vi "SLM_Control_Sample.vi"() -> ()   [LabVIEW 2018]
panel:
  in  "STOP button":bool
  out "Dffraction image":picture caption="Diffraction image"
  out "LG Beam image":picture
  out "Cylindrical lense image":picture caption="Cylindrical Lens image"
  out "Axicon image":picture
  out "Target image":picture
  out "Correction image":picture
  out "CGH image":picture caption="Tiled CGH image / Target image"
  out "Fresnel Lens image":picture
  out "2nd Display(LCOS) image":picture
  in  "?":T1(tab)
  in  "CGH  ON / OFF":bool=TRUE
  in  "LCOS type":string(combo)="X15223 series"
  in  "Corection image address":path
  in  "Target image address":path
  in  "Repetition Number":u32=100
  in  "Slip":i32
  in  "Cylindrical Lens":bool=TRUE
  in  "Cylindrical Focus/mm":i32=1000
  in  "WaveFront":bool=TRUE
  in  "Fresnel Lens":bool=TRUE
  in  "LUT":bool
  in  "2π Signal Level (0-255)":u8=210
  in  "Fresnel Focus/mm":i32=1000
  in  "Wave length/nm":u32=532
  out "Wave length/nm":u32=532
  in  "Mode Select":enum32{"Row", "Column"}(radio)
  in  "Rotation degree":dbl
  in  "Axicon Lens":bool=TRUE
  in  "Top level / πrad.":dbl=4.0
  in  "LG Beam":bool=TRUE
  in  "m":u32=1
  in  "p":u32=1
  in  "Diffraction":bool=TRUE
  in  "Mode Select2":enum32{"Row", "Column"}(radio)
  in  "gradation width":u32=1
  in  "gradation number":u32=2
  in  "Flip image":i32(listbox)
  in  "Beam size / mm":dbl
  in  "Additional phase mask (2πrad. at 0-255level) 2":path
  in  "Additional phase combination mode\nComplex amplitude / Amplitude 2":bool
  in  "Save 2nd Display image button":bool
  in  "Additional phase combination mode\nComplex amplitude / Amplitude 1":bool=TRUE
  in  "Monitor mumber":i32=2
  in  "Y PixelShift":i32
  in  "X PixelShift":i32
  in  "Additional phase mask (2πrad. at 0-255level) 1":path
  in  "Coef._2":bool=TRUE
  in  "Coef._2":dbl(slide)=1.0 scale=-10.0..10.0
  in  "m_2":i32=1
  in  "n_2":i32=1
  in  "diameter / mm":dbl=10.0 min=1.0
  in  "Coef._1":dbl(slide)=1.0 scale=-10.0..10.0
  in  "Zernike":bool=TRUE
  out "Zernike":picture caption="Zernike image"
  in  "n_1":i32=1
  in  "m_1":i32=-1
  in  "Coef._1":bool=TRUE
  # "Sample code for\nLabVIEW"
  # "Basic Setting Parameter"
  # "LCOS-SLM"
  # "If a null address was input , all 0 pattern will appear."
  # "Target image"
  # "Corection"
  # "CGH"
  # "LCOS display settings"
  # "After press the STOP button, the BMP data save dialog will open."
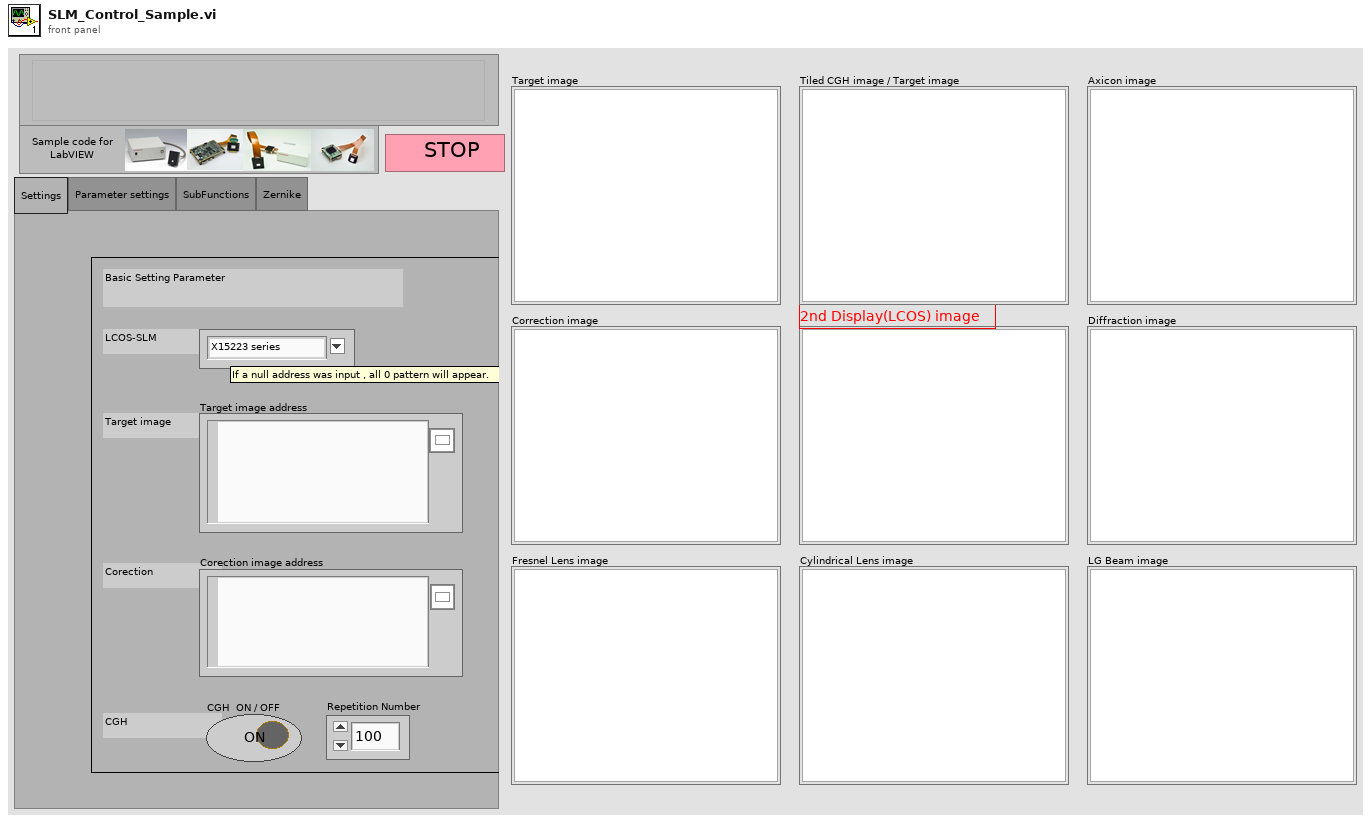
[diagram p1: front panel]
types:
  T1 = enum32{"Settings", "Parameter settings", "SubFunctions", "Zernike"}
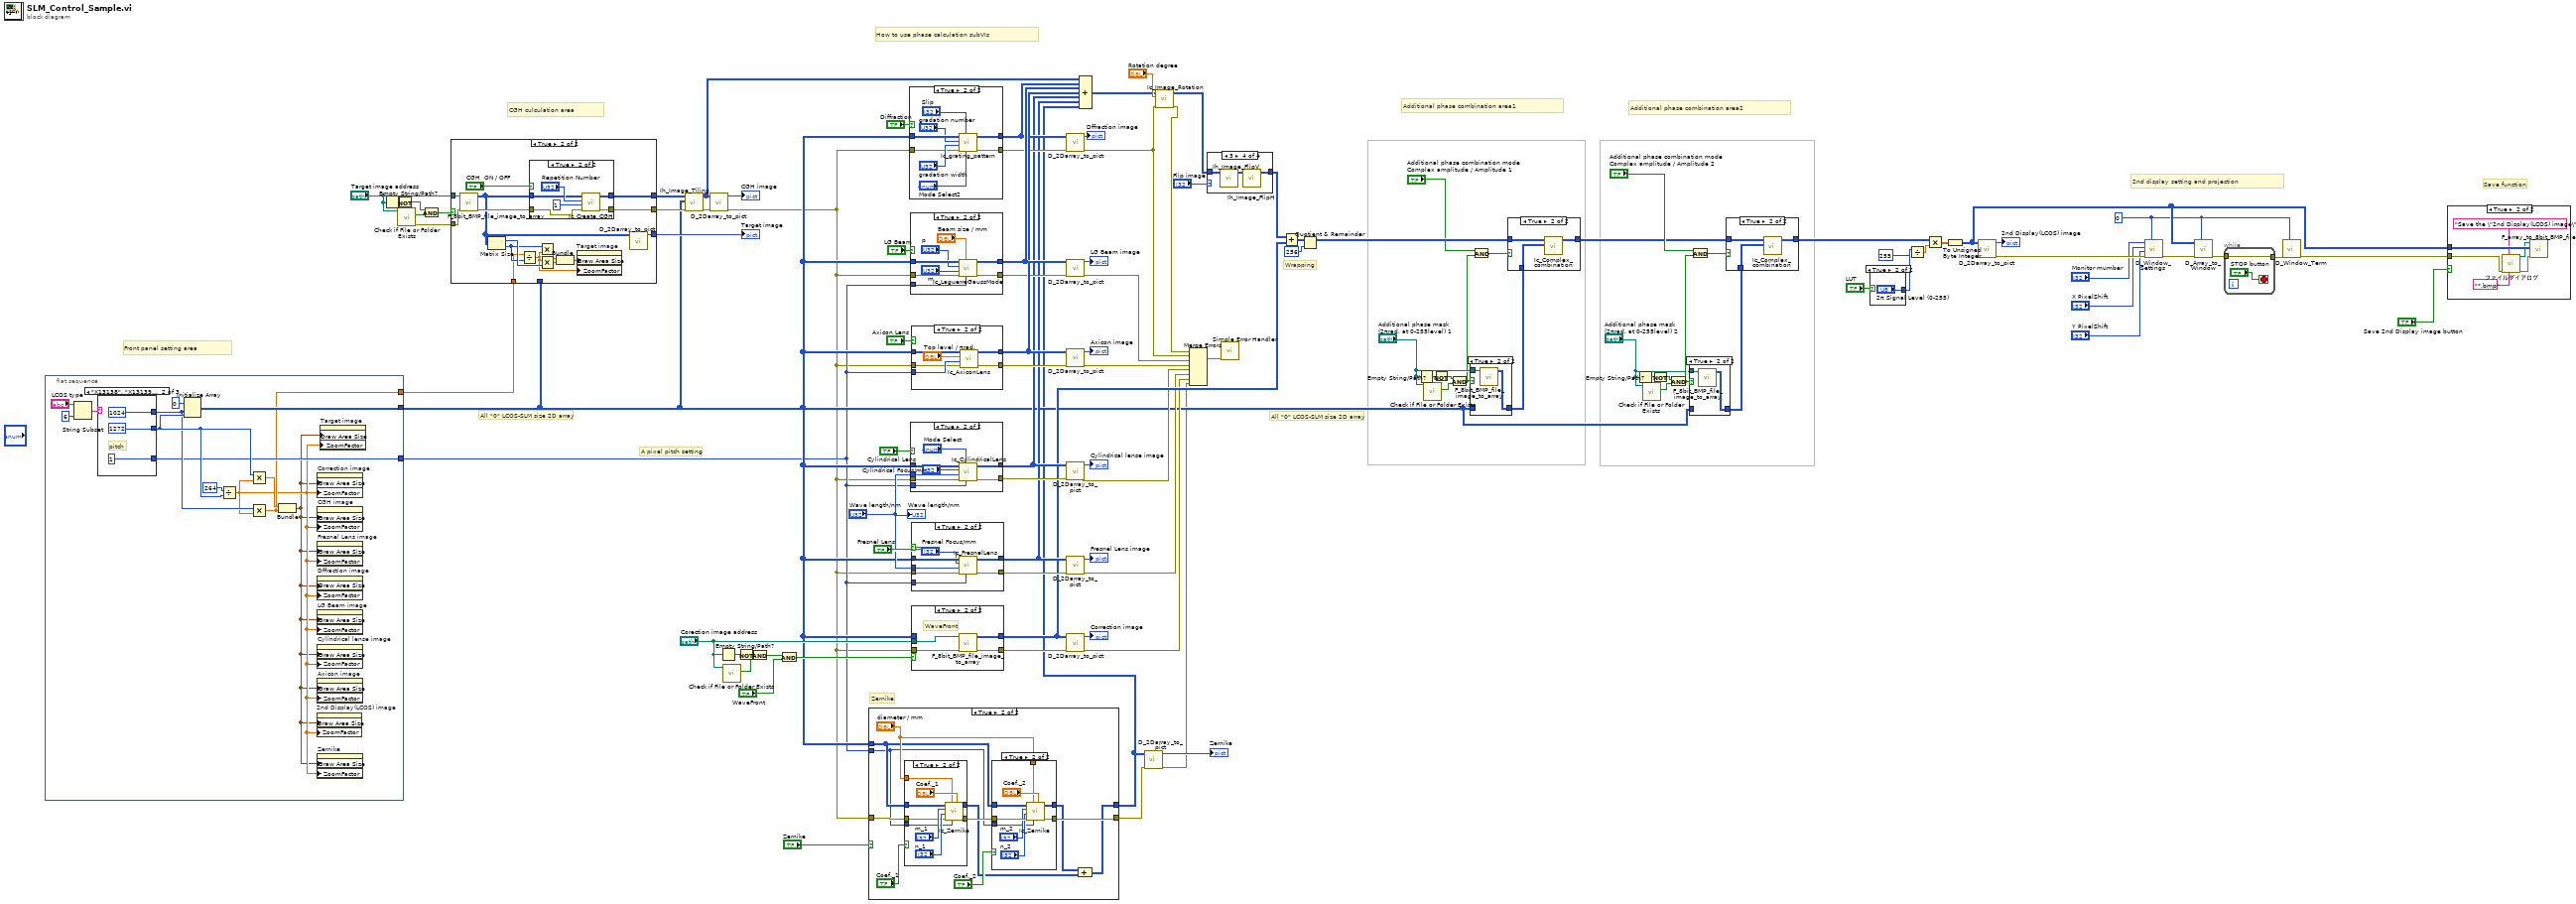
[diagram p0: block diagram]
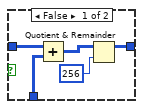
[diagram p6: hidden frame]
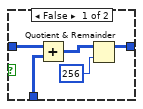
[diagram p8: hidden frame]
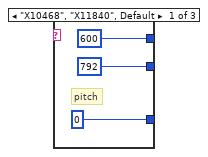
[diagram p10: hidden frame]
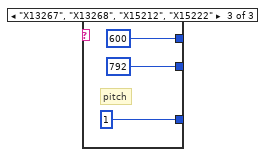
[diagram p11: hidden frame]
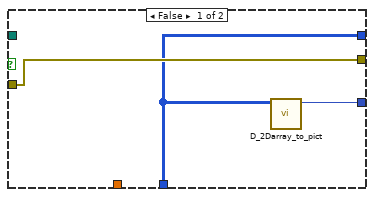
[diagram p12: hidden frame]
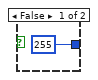
[diagram p19: hidden frame]
diagram:
  w23 = 0 ("Window Number (0...15)")
  # "Zernike"
  # "All \"0\" LCOS-SLM size 2D array"
  # "Save function"
  # "All \"0\" LCOS-SLM size 2D array"
  # "A pixel pitch setting"
  # "How to use phase calculation subVIs"
  # "CGH culculation area"
  # "Front panel setting area"
  # "2nd display setting and projection"
  # "Additional phase combination area2"
  # "Additional phase combination area1"
  # "Wrapping"
  n1 = flat-sequence {
    tunnel: [w108] -> w8
    tunnel: [w107] -> w7
    tunnel: [w106] -> w10
    frame #0 {
      n2 = String Subset(string="LCOS type", length (rest)=6 ("長さ（残り）")) -> (substring=w113:string)  [unwired: 1 in]
      n3 = case shown="\"X13138\", \"X13139\", \"X15213\", \"X15223\"" w113 {
        tunnel: [600 1024 600] -> w109
        tunnel: [792 1272 792] -> w110
        tunnel: [0 1 1] -> w107
        frame "X10468", "X11840", Default {
          # "pitch"
        }
        frame "X13138", "X13139", "X15213", "X15223" {
          # "pitch"
        }
        frame "X13267", "X13268", "X15212", "X15222" {
          # "pitch"
        }
      }
      n4 = Initialize Array(u8 0 ("要素"), w109, w110) -> (w108:u8[][])
      n5 = Divide(x=264, y=w110) -> (x/y=w105:dbl)
      n6 = Multiply(x=w110, y=w105) -> (x*y=w116:dbl)
      n7 = Multiply(x=w109, y=w105) -> (x*y=w106:dbl)
      n8 = Bundle(w116, w106) -> (w104:cluster{dbl, dbl})  [unwired: 1 in]
      n9 = property on="2nd Display(LCOS) image" class="Pict"("Draw Area Size"=w104, "ZoomFactor"=w105) -> ()  [unwired: 2 in, 2 out]
      n10 = property on="Correction image" class="Pict"("Draw Area Size"=w104, "ZoomFactor"=w105) -> ()  [unwired: 2 in, 2 out]
      n11 = property on="CGH image" class="Pict"("Draw Area Size"=w104, "ZoomFactor"=w105) -> ()  [unwired: 2 in, 2 out]
      n12 = property on="Fresnel Lens image" class="Pict"("Draw Area Size"=w104, "ZoomFactor"=w105) -> ()  [unwired: 2 in, 2 out]
      n13 = property on="Dffraction image" class="Pict"("Draw Area Size"=w104, "ZoomFactor"=w105) -> ()  [unwired: 2 in, 2 out]
      n14 = property on="LG Beam image" class="Pict"("Draw Area Size"=w104, "ZoomFactor"=w105) -> ()  [unwired: 2 in, 2 out]
      n15 = property on="Cylindrical lense image" class="Pict"("Draw Area Size"=w104, "ZoomFactor"=w105) -> ()  [unwired: 2 in, 2 out]
      n16 = property on="Axicon image" class="Pict"("Draw Area Size"=w104, "ZoomFactor"=w105) -> ()  [unwired: 2 in, 2 out]
      n17 = property on="Zernike" class="Pict"("Draw Area Size"=w104, "ZoomFactor"=w105) -> ()  [unwired: 2 in, 2 out]
      n18 = property on="Target image" class="Pict"("Draw Area Size"=w104, "ZoomFactor"=w105) -> ()  [unwired: 2 in, 2 out]
    }
  }
  n19 = Empty String/Path?(string/path="Target image address") -> (empty?=w79:bool)
  n20 = Not(x=w79) -> (.not. x?=w78:bool)
  n21 = call <vilib>:"Check if File or Folder Exists.vi"("path"="Target image address") -> ("error out"=w63:errorcluster, "file or folder exists?"=w76:bool)  [unwired: 8 in, 1 out]
  n22 = And(x=w78, y=w76) -> (x .and. y?=w77:bool)
  n23 = case shown="TRUE" w77 {
    tunnel: [w127 w142] -> w64
    tunnel: "Target image address" -> [_ w143]
    tunnel: w8 -> [w127 _]
    tunnel: w63 -> [w128 w140]
    tunnel: [w128 w138] -> w62
    tunnel: w10 -> [_ w131]
    tunnel: [w126 w130] -> w9
    frame False {
      n24 = call "D_2Darray_to_pict.vi"("2D array in"=w127) -> ("gray scale picture out"=w126:picture)  [unwired: 9 in, 1 out]
    }
    frame True {
      n25 = call "F_8bit_BMP_file_image_to_array.vi"("error in (no error)"=w140, "path to 8-bit BMP file"=w143) -> ("error out"=w139:errorcluster, "2D array out"=w129:u8[][])  [unwired: 8 in]
      n26 = Matrix Size(0:w129) -> (1:w136:i32, 2:w134:i32)
      n27 = Divide(x=w131, y=w134) -> (x/y=w132:dbl)
      n28 = case shown="TRUE" "CGH  ON / OFF" {
        tunnel: [w145 w150] -> w142
        tunnel: w129 -> [w145 w149]
        tunnel: w139 -> [w144 w147]
        tunnel: [w144 w146] -> w138
        frame False {
        }
        frame True {
          n29 = call "Ic_Create_CGH.vi"("2D array in"=w149, "Repetition Number"="Repetition Number", "progressBarOFF_0_ON_1"=u8 1, "error in (no error)"=w147) -> ("2D array out"=w150:u8[][], "error out"=w146:errorcluster)  [unwired: 5 in]
        }
      }
      n30 = Multiply(x=w134, y=w132) -> (x*y=w135:dbl)
      n31 = Multiply(x=w132, y=w136) -> (x*y=w137:dbl)
      n32 = Bundle(w135, w137) -> (w133:cluster{dbl, dbl})  [unwired: 1 in]
      n33 = property on="Target image" class="Pict"("Draw Area Size"=w133, "ZoomFactor"=w132) -> ()  [unwired: 2 in, 2 out]
      n34 = call "D_2Darray_to_pict.vi"("2D array in"=w129) -> ("gray scale picture out"=w130:picture)  [unwired: 9 in, 1 out]
    }
  }
  "Target image" <- w9
  n35 = call "Ih_Image_Tiling.vi"("error in (no error)"=w62, "2D array in (LCOS size buf)"=w8, "2D array in"=w64) -> ("error out"=w61:errorcluster, "2D array out"=w43:u8[][])  [unwired: 7 in]
  n36 = call "D_2Darray_to_pict.vi"("error in (no error)"=w61, "2D array in"=w43) -> ("error out"=w5:errorcluster, "gray scale picture out"=→"CGH image":picture)  [unwired: 8 in]
  n37 = Empty String/Path?(string/path="Corection image address") -> (empty?=w95:bool)
  n38 = call <vilib>:"Check if File or Folder Exists.vi"("path"="Corection image address") -> ("file or folder exists?"=w97:bool)  [unwired: 8 in, 2 out]
  n39 = Not(x=w95) -> (.not. x?=w96:bool)
  n40 = And(x=w96, y=w97) -> (x .and. y?=w92:bool)
  n41 = And(x=w92, y="WaveFront") -> (x .and. y?=w90:bool)
  n42 = case shown="TRUE" "Zernike" {
    tunnel: w8 -> [w153 w158]
    tunnel: w7 -> [_ w157]
    tunnel: [w153 w154] -> w1
    tunnel: w5 -> [w152 w164]
    tunnel: [w152 w162] -> w4
    frame False {
    }
    frame True {
      n43 = case shown="TRUE" "Coef._1" {
        tunnel: w158 -> [w177 w186]
        tunnel: w157 -> [_ w178]
        tunnel: w164 -> [w176 w183]
        tunnel: [w176 w181] -> w163
        tunnel: "diameter / mm" -> [_ w180]
        tunnel: [w177 w179] -> w155
        frame False {
        }
        frame True {
          n44 = call "Ic_Zernike.vi"("Coeff"="Coef._1", "Pixel Pitch 0:20um_or_ 1:12.5um"=w178, "diameter / mm"=w180, "error in (no error)"=w183, "n"="n_1", "m"="m_1", "2D array in (LCOS size buf)"=w186) -> ("error out"=w181:errorcluster, "2D array out"=w179:u8[][])  [unwired: 3 in]
        }
      }
      n45 = case shown="TRUE" "Coef._2" {
        tunnel: w163 -> [w165 w175]
        tunnel: [w165 w174] -> w162
        tunnel: [w166 w172] -> w156
        tunnel: w158 -> [w166 w171]
        tunnel: "diameter / mm" -> [_ w168]
        tunnel: w157 -> [_ w167]
        frame False {
        }
        frame True {
          n46 = call "Ic_Zernike.vi"("Coeff"="Coef._2", "Pixel Pitch 0:20um_or_ 1:12.5um"=w167, "diameter / mm"=w168, "error in (no error)"=w175, "n"="n_2", "m"="m_2", "2D array in (LCOS size buf)"=w171) -> ("error out"=w174:errorcluster, "2D array out"=w172:u8[][])  [unwired: 3 in]
        }
      }
      n47 = Compound Arithmetic op=ADD(w156, w155) -> (w154:u8[][])
    }
  }
  n48 = case shown="TRUE" "Diffraction" {
    tunnel: w8 -> [w188 w196]
    tunnel: [w188 w192] -> w65
    tunnel: w5 -> [w187 w191]
    tunnel: [w187 w190] -> w57
    frame False {
    }
    frame True {
      n49 = call "Ic_grating_pattern.vi"("Row:0 or column:1"="Mode Select2", "Slip_factor"="Slip", "error in (no error)"=w191, "gradation width"="gradation width", "gradation number"="gradation number", "2D array in (LCOS size buf)"=w196) -> ("error out"=w190:errorcluster, "2D array out"=w192:u8[][])  [unwired: 4 in]
    }
  }
  n50 = case shown="TRUE" "LG Beam" {
    tunnel: w8 -> [w198 w206]
    tunnel: [w198 w205] -> w74
    tunnel: w7 -> [_ w202]
    tunnel: w5 -> [w197 w201]
    tunnel: [w197 w200] -> w56
    frame False {
    }
    frame True {
      n51 = call "Ic_LaguerreGaussMode.vi"("Pixel Pitch 0:20um_or_ 1:12.5um"=w202, "Beam size / mm"="Beam size / mm", "error in (no error)"=w201, "m :azimuthal index"="m", "p :radial index"="p", "2D array in (LCOS size buf)"=w206) -> ("error out"=w200:errorcluster, "2D array out"=w205:u8[][])  [unwired: 4 in]
    }
  }
  n52 = case shown="TRUE" "Cylindrical Lens" {
    tunnel: "Wave length/nm" -> [_ w214]
    tunnel: [w208 w216] -> w40
    tunnel: w8 -> [w208 w213]
    tunnel: w5 -> [w207 w212]
    tunnel: [w207 w211] -> w58
    tunnel: w7 -> [_ w209]
    frame False {
    }
    frame True {
      n53 = call "Ic_CylindricalLens.vi"("Pixel Pitch 0:20um_or_ 1:12.5um"=w209, "Mode Select"="Mode Select", "error in (no error)"=w212, "Wave Length / nm"=w214, "Cylindrical Focus / mm"="Cylindrical Focus/mm", "2D array in (LCOS size buf)"=w213) -> ("error out"=w211:errorcluster, "2D array out"=w216:u8[][])  [unwired: 4 in]
    }
  }
  n54 = case shown="TRUE" "Axicon Lens" {
    tunnel: w8 -> [w218 w224]
    tunnel: [w218 w223] -> w72
    tunnel: w7 -> [_ w221]
    tunnel: w5 -> [w217 w220]
    tunnel: [w217 w219] -> w55
    frame False {
    }
    frame True {
      n55 = call "Ic_AxiconLens.vi"("error in (no error)"=w220, "Pixel Pitch 0:20um_or_ 1:12.5um"=w221, "Top level / πrad."="Top level / πrad.", "2D array in (LCOS size buf)"=w224) -> ("error out"=w219:errorcluster, "2D array out"=w223:u8[][])  [unwired: 6 in]
    }
  }
  n56 = case shown="TRUE" "Fresnel Lens" {
    tunnel: "Wave length/nm" -> [_ w230]
    tunnel: w7 -> [_ w231]
    tunnel: w8 -> [w226 w233]
    tunnel: [w226 w232] -> w39
    tunnel: w5 -> [w225 w229]
    tunnel: [w225 w228] -> w59
    frame False {
    }
    frame True {
      n57 = call "Ic_FresnelLens.vi"("Pixel Pitch 0:20um_or_ 1:12.5um"=w231, "error in (no error)"=w229, "Wave length / nm"=w230, "Focus / mm"="Fresnel Focus/mm", "2D array in (LCOS size buf)"=w233) -> ("error out"=w228:errorcluster, "2D array out"=w232:u8[][])  [unwired: 5 in]
    }
  }
  n58 = case shown="TRUE" w90 {
    tunnel: "Corection image address" -> [_ w238]
    tunnel: [w235 w239] -> w38
    tunnel: w8 -> [w235 _]
    tunnel: w5 -> [w234 w237]
    tunnel: [w234 w236] -> w60
    frame False {
    }
    frame True {
      # "WaveFront"
      n59 = call "F_8bit_BMP_file_image_to_array.vi"("error in (no error)"=w237, "path to 8-bit BMP file"=w238) -> ("error out"=w236:errorcluster, "2D array out"=w239:u8[][])  [unwired: 8 in]
    }
  }
  n60 = call "D_2Darray_to_pict.vi"("error in (no error)"=w57, "2D array in"=w65) -> ("error out"=w52:errorcluster, "gray scale picture out"=→"Dffraction image":picture)  [unwired: 8 in]
  n61 = call "D_2Darray_to_pict.vi"("error in (no error)"=w56, "2D array in"=w74) -> ("error out"=w53:errorcluster, "gray scale picture out"=→"LG Beam image":picture)  [unwired: 8 in]
  n62 = call "D_2Darray_to_pict.vi"("error in (no error)"=w55, "2D array in"=w72) -> ("error out"=w54:errorcluster, "gray scale picture out"=→"Axicon image":picture)  [unwired: 8 in]
  n63 = call "D_2Darray_to_pict.vi"("error in (no error)"=w58, "2D array in"=w40) -> ("error out"=w37:errorcluster, "gray scale picture out"=→"Cylindrical lense image":picture)  [unwired: 8 in]
  n64 = call "D_2Darray_to_pict.vi"("error in (no error)"=w59, "2D array in"=w39) -> ("error out"=w36:errorcluster, "gray scale picture out"=→"Fresnel Lens image":picture)  [unwired: 8 in]
  n65 = call "D_2Darray_to_pict.vi"("error in (no error)"=w60, "2D array in"=w38) -> ("error out"=w35:errorcluster, "gray scale picture out"=→"Correction image":picture)  [unwired: 8 in]
  n66 = Compound Arithmetic op=ADD(w43, w65, w74, w72, w40, w39, w1) -> (w82:u8[][])
  n67 = call "D_2Darray_to_pict.vi"("error in (no error)"=w4, "2D array in"=w1) -> ("error out"=w3:errorcluster, "gray scale picture out"=→"Zernike":picture)  [unwired: 8 in]
  n68 = call "Ic_Image_Rotation.vi"("error in (no error)"=w52, "degree"="Rotation degree", "2D array in"=w82) -> ("error out"=w51:errorcluster, "2D array out"=w87:u8[][])  [unwired: 7 in]
  n69 = Merge Errors(w51, w52, w53, w54, w37, w36, w35, w3) -> (w50:errorcluster)
  n70 = case shown="3" "Flip image" {
    tunnel: w87 -> [w240 w242 w244 w245]
    tunnel: [w240 w241 w243 w246] -> w81
    frame 0, Default {
    }
    frame 1 {
      n71 = call "Ih_Image_FlipV.vi"("2D array in"=w242) -> ("Flip V 2D array out"=w241:u32[][])  [unwired: 10 in]
    }
    frame 2 {
      n72 = call "Ih_Image_FlipH.vi"("2D array in"=w244) -> ("Flip H 2D array out"=w243:u32[][])  [unwired: 10 in]
    }
    frame 3 {
      n73 = call "Ih_Image_FlipV.vi"("2D array in"=w245) -> ("Flip V 2D array out"=w247:u32[][])  [unwired: 10 in]
      n74 = call "Ih_Image_FlipH.vi"("2D array in"=w247) -> ("Flip H 2D array out"=w246:u32[][])  [unwired: 10 in]
    }
  }
  n75 = call <vilib>:"Simple Error Handler.vi"("error in (no error)"=w50) -> ()  [unwired: 4 in, 5 out]
  n76 = Add(x=w81, y=w38) -> (x+y=w42:u32[][])
  n77 = Quotient & Remainder(x=w42, y=256) -> (x-y*floor(x/y)=w34:u32[][])  [unwired: 1 out]
  n78 = Empty String/Path?(string/path="Additional phase mask (2πrad. at 0-255level) 1") -> (empty?=w28:bool)
  n79 = call <vilib>:"Check if File or Folder Exists.vi"("path"="Additional phase mask (2πrad. at 0-255level) 1") -> ("file or folder exists?"=w32:bool)  [unwired: 8 in, 2 out]
  n80 = Not(x=w28) -> (.not. x?=w31:bool)
  n81 = And(x=w31, y=w32) -> (x .and. y?=w26:bool)
  n82 = case shown="TRUE" w26 {
    tunnel: "Additional phase mask (2πrad. at 0-255level) 1" -> [_ w250]
    tunnel: w8 -> [w248 _]
    tunnel: [w248 w249] -> w29
    frame False {
    }
    frame True {
      n83 = call "F_8bit_BMP_file_image_to_array.vi"("path to 8-bit BMP file"=w250) -> ("2D array out"=w249:u8[][])  [unwired: 9 in, 1 out]
    }
  }
  n84 = And(x="Additional phase combination mode\nComplex amplitude / Amplitude 1", y=w26) -> (x .and. y?=w25:bool)
  n85 = case shown="TRUE" w25 {
    tunnel: w34 -> [w255 w258]
    tunnel: [w251 w256] -> w13
    tunnel: w29 -> [w254 w257]
    frame False {
      n86 = Add(x=w255, y=w254) -> (x+y=w252:u32[][])
      n87 = Quotient & Remainder(x=w252, y=256) -> (x-y*floor(x/y)=w251:u32[][])  [unwired: 1 out]
    }
    frame True {
      n88 = call "Ic_Complex_combination.vi"("2D array in 2"=w257, "2D array in"=w258) -> ("2D array out"=w256:u8[][])  [unwired: 9 in]
    }
  }
  n89 = Empty String/Path?(string/path="Additional phase mask (2πrad. at 0-255level) 2") -> (empty?=w19:bool)
  n90 = call <vilib>:"Check if File or Folder Exists.vi"("path"="Additional phase mask (2πrad. at 0-255level) 2") -> ("file or folder exists?"=w22:bool)  [unwired: 8 in, 2 out]
  n91 = Not(x=w19) -> (.not. x?=w21:bool)
  n92 = And(x=w21, y=w22) -> (x .and. y?=w18:bool)
  n93 = case shown="TRUE" w18 {
    tunnel: "Additional phase mask (2πrad. at 0-255level) 2" -> [_ w261]
    tunnel: w8 -> [w259 _]
    tunnel: [w259 w260] -> w20
    frame False {
    }
    frame True {
      n94 = call "F_8bit_BMP_file_image_to_array.vi"("path to 8-bit BMP file"=w261) -> ("2D array out"=w260:u8[][])  [unwired: 9 in, 1 out]
    }
  }
  n95 = And(x="Additional phase combination mode\nComplex amplitude / Amplitude 2", y=w18) -> (x .and. y?=w17:bool)
  n96 = case shown="TRUE" w17 {
    tunnel: w13 -> [w266 w269]
    tunnel: [w262 w267] -> w14
    tunnel: w20 -> [w265 w268]
    frame False {
      n97 = Add(x=w266, y=w265) -> (x+y=w263:u32[][])
      n98 = Quotient & Remainder(x=w263, y=256) -> (x-y*floor(x/y)=w262:u32[][])  [unwired: 1 out]
    }
    frame True {
      n99 = call "Ic_Complex_combination.vi"("2D array in 2"=w268, "2D array in"=w269) -> ("2D array out"=w267:u8[][])  [unwired: 9 in]
    }
  }
  n100 = case shown="TRUE" "LUT" {
    tunnel: [255 ("2π Signal Level (0-255)") "2π Signal Level (0-255)"] -> w100
    frame False {
    }
    frame True {
    }
  }
  n101 = Divide(x=w100, y=255) -> (x/y=w101:dbl)
  n102 = Multiply(x=w14, y=w101) -> (x*y=w99:dbl[][])
  n103 = To Unsigned Byte Integer(number=w99) -> (unsigned 8bit integer=w47:u8[][])
  n104 = call "D_2Darray_to_pict.vi"("2D array in"=w47) -> ("error out"=w49:errorcluster, "gray scale picture out"=→"2nd Display(LCOS) image":picture)  [unwired: 9 in]
  n105 = call "D_Window_Settings.vi"("Window Number (0...15)"=w23, "error in (no error)"=w49, "YPixelShift"="Y PixelShift", "XPixelShift"="X PixelShift", "Monitor mumber"="Monitor mumber") -> ("error out"=w48:errorcluster)  [unwired: 6 in]
  n106 = call "D_Array_to_Window.vi"("Window Number (0...15)"=w23, "error in (no error)"=w48, "Image Pixels (U8)"=w47) -> ("error out"=w12:errorcluster)  [unwired: 8 in]
  n107 = while {
    tunnel: w12 -> [w273]
    tunnel: [w273] -> w11
    stop <- "STOP button" stop-if-true
  }
  n108 = call "D_Window_Term.vi"("Window Number (0...15)"=w23, "error in (no error)"=w11) -> ("error out"=w24:errorcluster)  [unwired: 9 in]
  n109 = case shown="TRUE" "Save 2nd Display image button" {
    tunnel: w24 -> [_ w275]
    tunnel: w47 -> [_ w279]
    frame False {
    }
    frame True {
      n110 = call "ファイルダイアログ"("prompt"="Save the \"2nd Display(LCOS) image\"", "error in"=w275, "pattern (all files)"="*.bmp") -> ("selected path"=w278:path, "error out"=w274:errorcluster)  [unwired: 9 in, 2 out]
      n111 = call "F_array_to_8bit_BMP_file.vi"("error in (no error)"=w274, "2D array in"=w279, "path to save BMP file"=w278) -> ()  [unwired: 8 in, 1 out]
    }
  }
  "Wave length/nm" <- "Wave length/nm"
